vi "InitMiscellaneous.vi"   [LabVIEW 2020]
doc: "This VI initializes miscellaneous devices such as the compressor and any decorations."
uses:
  <vilib>/Rock Robotics/WPI/Utilities/WPI_GetSetVariantRefNum.vi
  refnums.vi
types:
  T1 = typedef "WPI_CompressorDevRef.ctl" = cluster{"DevStatus":errorcluster, "Pneumatics Control Module":u8}
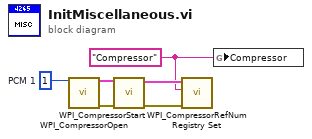
[diagram p0: block diagram]
diagram:
  w1 = "Compressor" ("refnum name")
  w2 = u8 1  # PCM 1
  n1 = call <vilib>:"WPI_CompressorOpen.vi"("Pneumatics device (def)"=w2) -> ("CompressorDevRef"=w5:T1, "error out"=w6:errorcluster)  [unwired: 13 in]
  n2 = call <vilib>:"WPI_CompressorStart.vi"("error in (no error)"=w6, "CompressorDevRef"=w5) -> ("error out"=w3:errorcluster, "CompressorDevRef"=w4:T1)  [unwired: 8 in]
  n3 = call <vilib>:"WPI_CompressorRefNum Registry Set.vi"("error in (no error)"=w3, "refnum name"=w1, "CompressorDevRef"=w4) -> ()  [unwired: 7 in, 2 out]
  n4 = global write "refnums.vi" "Compressor"(w1) -> ()
